vi "Periodic Tasks.vi"(8 "error in":errorcluster) -> (0 "error out":errorcluster)   [LabVIEW 2020]
doc: "This VI runs in parallel to other tasks. It can contain as many user-defined periodic loops as you need. These can carry out PID or other sorts of timed response."
uses:
  <vilib>/Rock Robotics/WPI/ThirdParty/Phoenix-LabVIEW/Motor Controller/Controls/CTRE_Phoenix_MotorControl_ControlMode.ctl
  <vilib>/Rock Robotics/WPI/Utilities/WPI_GetSetVariantRefNum.vi
  Robot Global Data.vi
  2018 Power Up/2018 Robot Project V.3.0/Robot Global Data V.3.0.vi
panel:
  out "Dart Run Speed":dbl
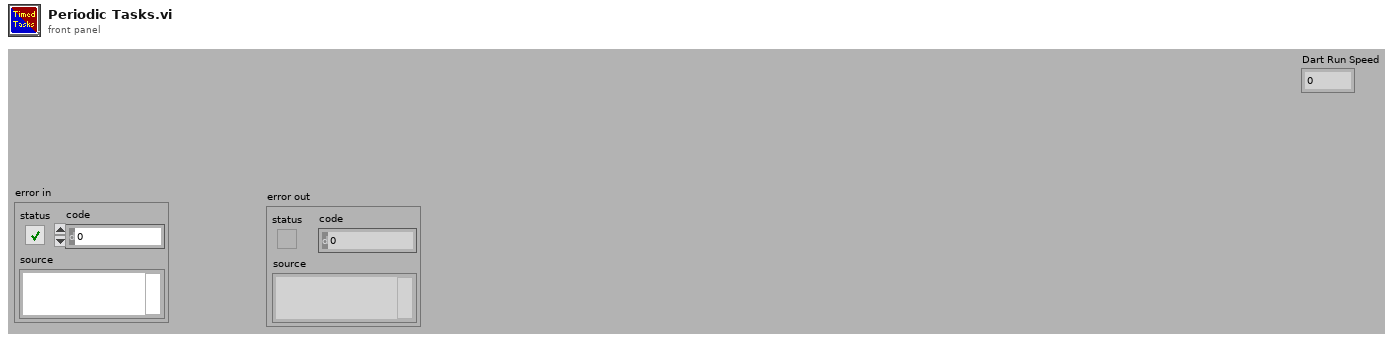
[diagram p1: front panel]
types:
  T1 = typedef "WPI_CounterDevRef.ctl" = cluster{"DevStatus":errorcluster, "CntIndex":T2}
  T2 = typedef "FPGA_CounterCtrSystemIndex.ctl" = enum8{"Ctr 0", "Ctr 1", "Ctr 2", "Ctr 3", "Ctr 4", "Ctr 5", "Ctr 6", "Ctr 7", "Invalid"}
  T3 = typedef "WPI_JoystickDevRef.ctl" = cluster{"Device":T4}
  T4 = typedef "WPI_JoystickDeviceEnum.ctl" = enum16{"USB 0", "USB 1", "USB 2", "USB 3", "USB 4", "USB 5"}
  T5 = typedef "WPI_ServoDeviceRef.ctl" = cluster{"DeviceStatus":errorcluster, "PWM Channel":T6, "DeadBand":T7}
  T6 = typedef "FPGA_DIOPWMChannel.ctl" = enum8{"PWM 0", "PWM 1", "PWM 2", "PWM 3", "PWM 4", "PWM 5", "PWM 6", "PWM 7", "PWM 8", "PWM 9", "PWM MXP 0", "PWM MXP 1", "PWM MXP 2", "PWM MXP 3", "PWM MXP 4", "PWM MXP 5", "PWM MXP 6", "PWM MXP 7", "PWM MXP 8", "PWM MXP 9", "Invalid"}
  T7 = typedef "WPI_PWMDeadband.ctl" = cluster{"Name":string, "maxPositivePwm":i32, "minPositivePwm":i32, "centerPwm":i32, "maxNegativePwm":i32, "minNegativePwm":i32, "angularRange":u16}
  T8 = typedef "WPI_PotentiometerDevRef.ctl" = cluster{"DevStatus":errorcluster, "Analog Channel":T9, "Invert Output":bool}
  T9 = typedef "FPGA_AIChannel.ctl" = enum8{"AI 0", "AI 1", "AI 2", "AI 3", "AI MXP 0", "AI MXP 1", "AI MXP 2", "AI MXP 3", "Invalid"}
  T10 = typedef "WPI_AnalogChannelDevRef.ctl" = cluster{"DevStatus":errorcluster, "Analog Channel":T9}
  T11 = typedef "WPI_DriverStationRobotMode2.ctl" = enum16{"Autonomous Disabled", "Autonomous Enabled", "Teleop Disabled", "Teleop Enabled", "Disconnected", "Finish", "Test Disabled", "Test Enabled", "Emergency Stopped"}
  T12 = typedef "WPI_MotorControlDeviceRef.ctl" = cluster{"DeviceStatus":errorcluster, "Type":T13, "PWM":cluster{"PWM Channel":T6, "DeadBand":T7}, "CAN":cluster{"Device Number":u8, "SetOutput VI Ref":variant, "GetOutput VI Ref":variant, "Enable VI Ref":variant, "Disable VI Ref":variant, "Data":variant}, "Invert":bool, "DIO PWM":cluster{"PWM \"Enable\" Channel":T6, "DIOChannel":T14, "PWM Rate":dbl}}
  T13 = typedef "WPI_MotorControlType.ctl" = enum16{"PWM", "CAN", "DIO PWM"}
  T14 = typedef "FPGA_DIOChannel.ctl" = enum8{"DIO 0", "DIO 1", "DIO 2", "DIO 3", "DIO 4", "DIO 5", "DIO 6", "DIO 7", "DIO 8", "DIO 9", "DIO MXP 0", "DIO MXP 1", "DIO MXP 2", "DIO MXP 3", "DIO MXP 4", "DIO MXP 5", "DIO MXP 6", "DIO MXP 7", "DIO MXP 8", "DIO MXP 9", "DIO MXP 10", "DIO MXP 11", "DIO MXP 12", "DIO MXP 13", "DIO MXP 14", "DIO MXP 15", "SPI Port CS1", "SPI Port CS2", "SPI Port CS3", "SPI Port MISO", "SPI Port MOSI", "Invalid"}
  T15 = typedef "CTRE_Phoenix_MotorControl_ControlMode.ctl" = u16
  T16 = cluster{"Pot. Voltage":dbl[], "Corresponding Inches":dbl[]}
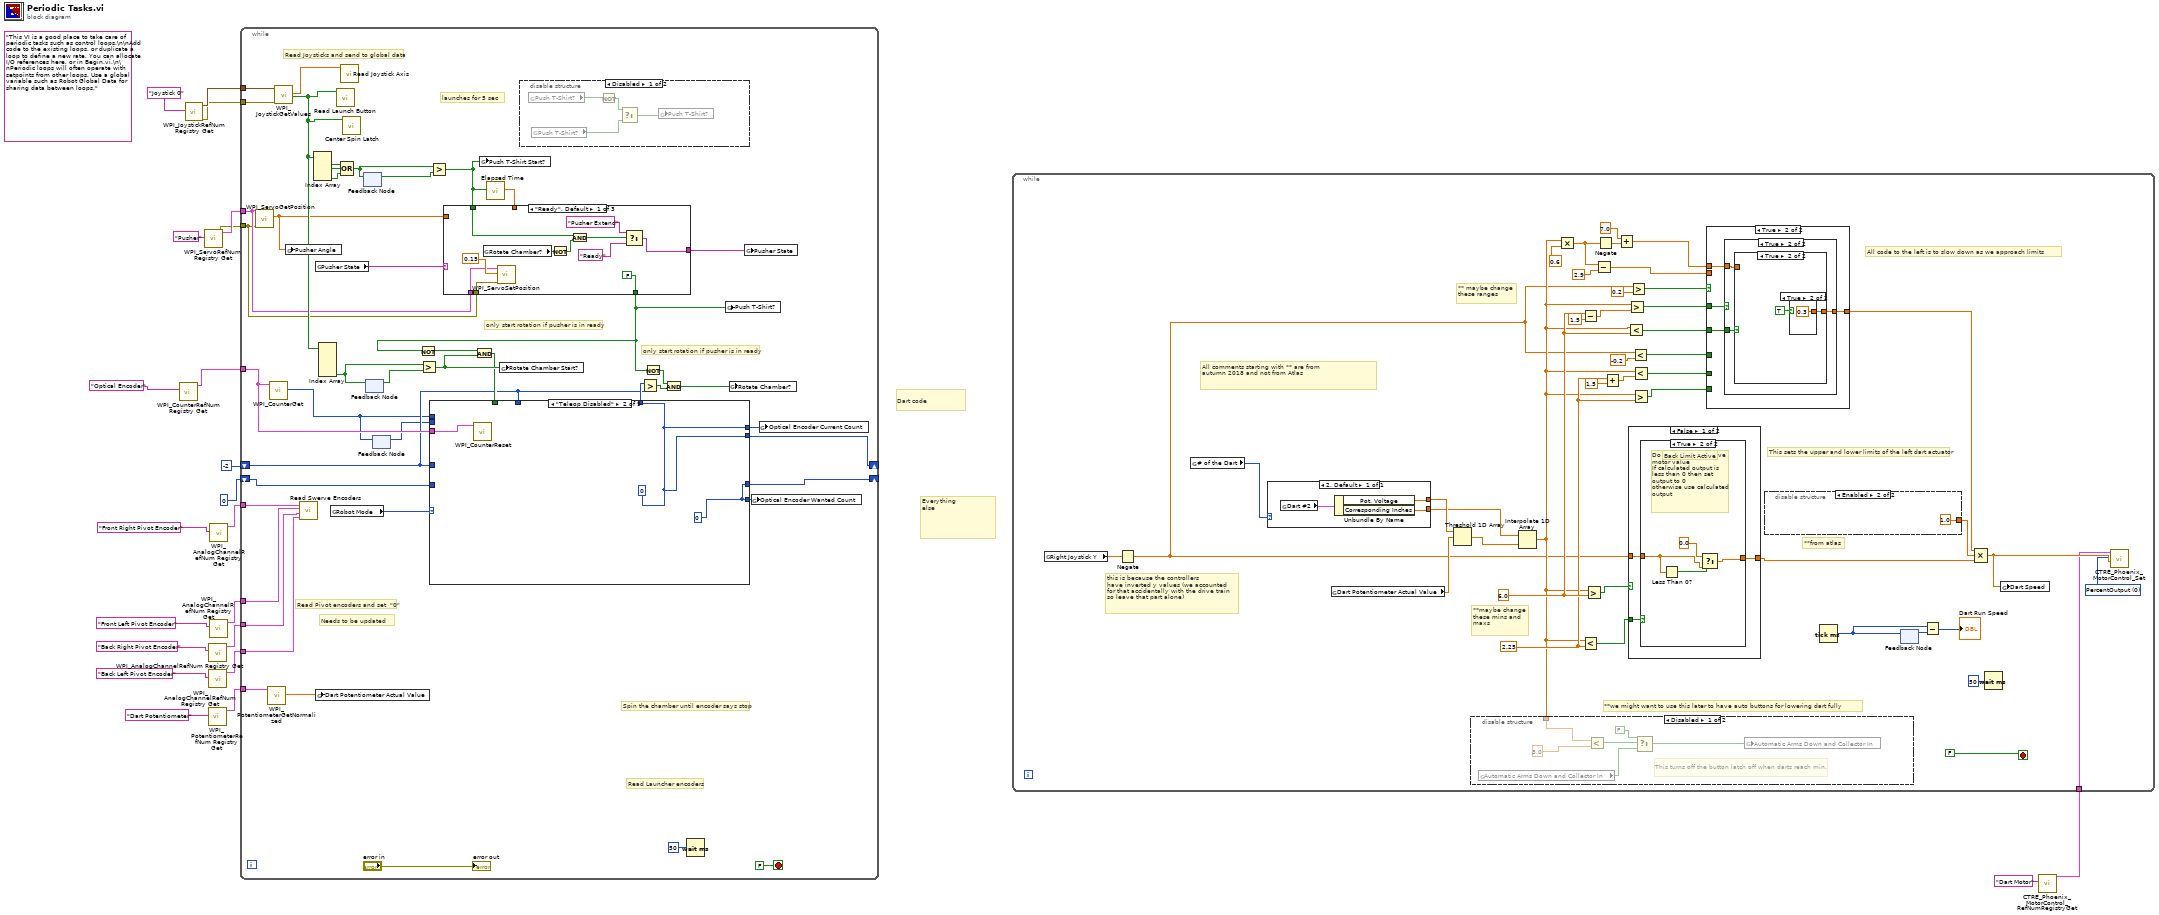
[diagram p0: block diagram]
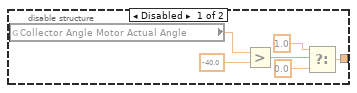
[diagram p2: hidden frame]
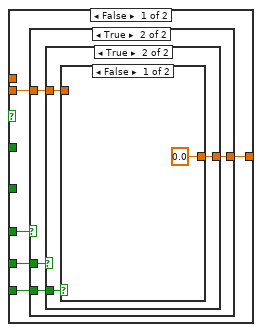
[diagram p4: hidden frame]
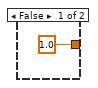
[diagram p5: hidden frame]
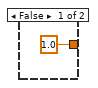
[diagram p6: hidden frame]
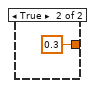
[diagram p7: hidden frame]
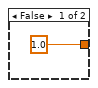
[diagram p8: hidden frame]
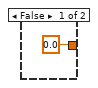
[diagram p9: hidden frame]
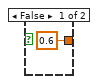
[diagram p10: hidden frame]
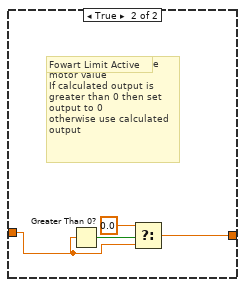
[diagram p12: hidden frame]
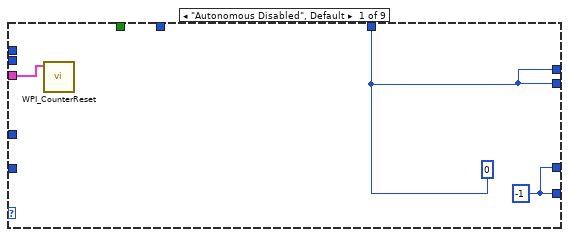
[diagram p13: hidden frame]
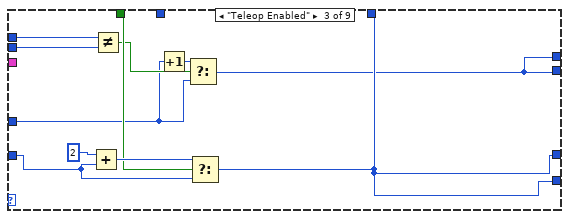
[diagram p14: hidden frame]
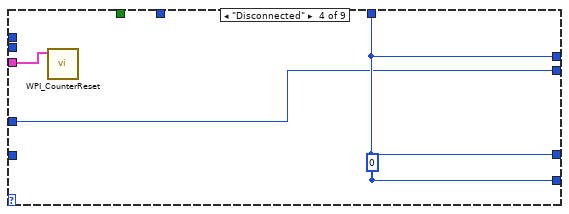
[diagram p15: hidden frame]
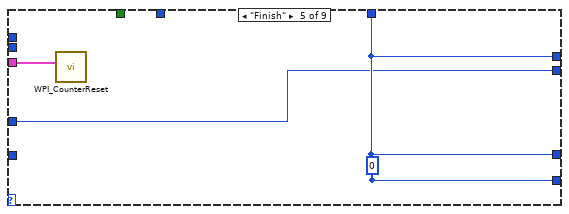
[diagram p16: hidden frame]
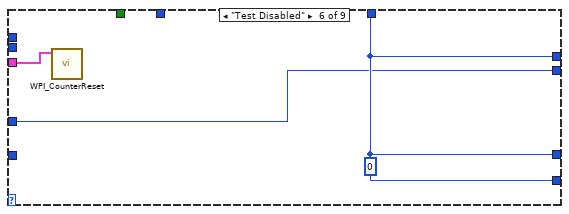
[diagram p17: hidden frame]
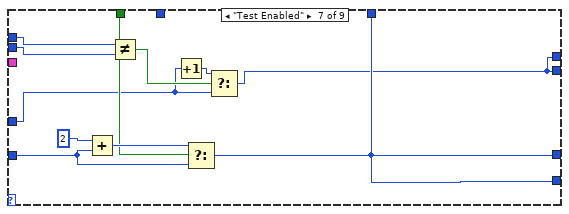
[diagram p18: hidden frame]
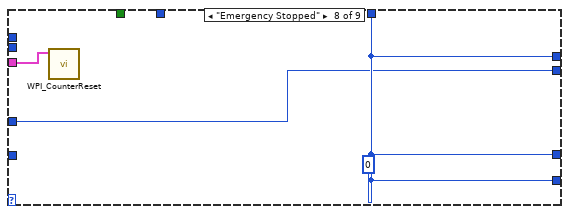
[diagram p19: hidden frame]
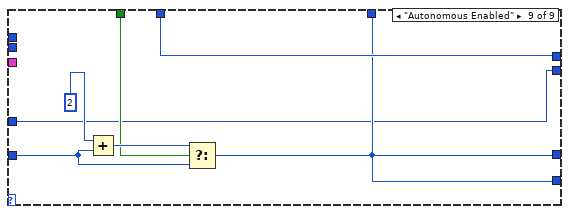
[diagram p20: hidden frame]
diagram:
  (unwired) "This VI is a good place to take care of periodic tasks such as control loops.\n\nAdd code to the existing loops, or duplicate a loop to define a new rate. You can allocate I/O references here, or in Begin.vi.\n\nPeriodic loops will often operate with setpoints from other loops. Use a global variable such as Robot Global Data for sharing data between loops."
  # "Everything\nelse"
  # "Dart code"
  n1 = call <vilib>:"WPI_CounterRefNum Registry Get.vi"("refnum name"="Optical Encoder") -> ("CounterDevRef"=w12:T1)  [unwired: 9 in, 1 out]
  n2 = call <vilib>:"WPI_JoystickRefNum Registry Get.vi"("refnum name"="Joystick 0") -> ("error out"=w20:errorcluster, "JoystickDevRef"=w21:T3)  [unwired: 9 in]
  n3 = call <vilib>:"WPI_ServoRefNum Registry Get.vi"("refnum name"="Pusher") -> ("error out"=w7:errorcluster, "ServoDeviceRef"=w8:T5)  [unwired: 9 in]
  n4 = call <vilib>:"WPI_PotentiometerRefNum Registry Get.vi"("refnum name"="Dart Potentiometer") -> ("PotDevRef"=w4:T8)  [unwired: 9 in, 1 out]
  n5 = call <vilib>:"WPI_AnalogChannelRefNum Registry Get.vi"("refnum name"="Back Right Pivot Encoder") -> ("AIDeviceRef"=w14:T10)  [unwired: 1 in, 9 out]
  n6 = call <vilib>:"WPI_AnalogChannelRefNum Registry Get.vi"("refnum name"="Back Left Pivot Encoder") -> ("AIDeviceRef"=w9:T10)  [unwired: 1 in, 9 out]
  n7 = call <vilib>:"WPI_AnalogChannelRefNum Registry Get.vi"("refnum name"="Front Left Pivot Encoder") -> ("AIDeviceRef"=w15:T10)  [unwired: 1 in, 9 out]
  n8 = call <vilib>:"WPI_AnalogChannelRefNum Registry Get.vi"("refnum name"="Front Right Pivot Encoder") -> ("AIDeviceRef"=w18:T10)  [unwired: 1 in, 9 out]
  n9 = while {
    tunnel: w21 -> [w66]
    tunnel: w20 -> [w65]
    tunnel: w18 -> [w61]
    tunnel: w15 -> [w60]
    tunnel: w14 -> [w59]
    tunnel: w12 -> [w27]
    shift-right: [w33] -> _
    shift-left: 0 -> [w29]
    tunnel: w9 -> [w57]
    tunnel: w8 -> [w51]
    tunnel: w7 -> [w50]
    tunnel: w4 -> [w41]
    shift-right: [w26] -> _
    shift-left: -2 -> [w25]
    stop <- FALSE stop-if-true
    # "only start rotation if pusher is in ready"
    # "only start rotation if pusher is in ready"
    # "Needs to be updated"
    # "launches for 5 sec"
    # "Read Launcher encoders"
    # "Read Pivot encoders and set  \"0\""
    # "Spin the chamber until encoder says stop"
    # "Read Joysticks and send to global data"
    n10 = call <vilib>:"WPI_ServoGetPosition.vi"("error in (no error)"=w50, "ServoDeviceRef"=w51) -> ("Position"=w52:dbl)  [unwired: 7 in, 2 out]
    n11 = call <vilib>:"WPI_PotentiometerGetNormalized.vi"("PotDevRef"=w41) -> ("Normalized Value"=w40:dbl)  [unwired: 8 in, 2 out]
    n12 = call <vilib>:"WPI_CounterGet.vi"("CounterDevRef in"=w27) -> ("Value"=w23:i32)  [unwired: 5 in, 5 out]
    n13 = call <vilib>:"WPI_JoystickGetValues.vi"("error in (no error)"=w65, "JoystickDevRef"=w66) -> ("Buttons"=w56:bool[], "Axes"=w62:dbl[])  [unwired: 5 in, 3 out]
    n14 = global write "Robot Global Data.vi" "Pusher Angle"(w52) -> ()
    n15 = call "Read Swerve Encoders.vi"("BL Ref"=w57, "BR Ref"=w59, "FL Ref"=w60, "FR Ref"=w61) -> ()  [unwired: 1 in]
    n16 = Index Array(array=w56) -> (element #1=w38:bool, element #2=w37:bool, element #4=w36:bool)  [unwired: 4 in, 1 out]
    n17 = global read "Robot Global Data.vi" "Pusher State"() -> (w54:string)
    n18 = global write "Robot Global Data.vi" "Dart Potentiometer Actual Value"(w40) -> ()
    n19 = Index Array(array=w56) -> (element #5=w39:bool)  [unwired: 5 in, 4 out]
    n20 = global read "Robot Global Data.vi" "Robot Mode"() -> (w34:T11)
    n21 = call "Read Launch Button.vi"("array"=w56) -> ()  [unwired: 11 in]
    n22 = call "Read Joystick Axis.vi"("Joystick 0"=w62) -> ()  [unwired: 11 in]
    n23 = Compound Arithmetic op=OR(w38, w37, w36) -> (w35:bool)
    n24 = call "Center Spin Latch.vi"("array"=w56) -> ()  [unwired: 11 in]
    n25 = feedback #1() -> (w55:bool)  [unwired: 1 in]
    n26 = feedback-in #1(w35) -> ()
    n27 = feedback-in #2(w39) -> ()
    n28 = feedback #2() -> (w58:bool)  [unwired: 1 in]
    n29 = feedback #3() -> (w24:i32)  [unwired: 1 in]
    n30 = feedback-in #3(w23) -> ()
    n31 = Greater?(x=w39, y=w58) -> (0:w42:bool)
    n32 = Greater?(x=w35, y=w55) -> (0:w49:bool)
    n33 = global write "Robot Global Data.vi" "Push T-Shirt Start?"(w49) -> ()
    n34 = call "Elapsed Time"("Reset"=w49) -> ("Elapsed Time (s)"=w48:dbl)  [unwired: 11 in, 7 out]
    n35 = case shown="\"Ready\", Default" w54 {
      tunnel: w49 -> [w121 _ _]
      tunnel: [w128 w139 w146] -> w53
      tunnel: w52 -> [_ _ _]
      tunnel: w51 -> [w124 w138 w147]
      tunnel: w50 -> [w125 w135 w145]
      tunnel: [FALSE TRUE TRUE] -> w43
      tunnel: w48 -> [_ w131 w141]
      frame "Ready", Default {
        n36 = global read "Robot Global Data.vi" "Rotate Chamber?"() -> (w123:bool)
        n37 = call <vilib>:"WPI_ServoSetPosition.vi"("error in (no error)"=w125, "Position"=0.15, "ServoDeviceRef"=w124) -> ()  [unwired: 7 in, 2 out]
        n38 = Not(x=w123) -> (.not. x?=w122:bool)
        n39 = And(x=w121, y=w122) -> (x .and. y?=w120:bool)
        n40 = Select(t="Pusher Extend", s=w120, f="Ready") -> (s? t:f=w128:string)
      }
      frame "Pusher Extend" {
        n41 = call <vilib>:"WPI_ServoSetPosition.vi"("error in (no error)"=w135, "Position"=0.9, "ServoDeviceRef"=w138) -> ()  [unwired: 7 in, 2 out]
        n42 = Greater Or Equal?(x=w131, y=5.0) -> (x >= y?=w132:bool)
        n43 = Select(t="Pusher Retract", s=w132, f="Pusher Extend") -> (s? t:f=w139:string)
      }
      frame "Pusher Retract" {
        n44 = call <vilib>:"WPI_ServoSetPosition.vi"("error in (no error)"=w145, "Position"=0.15, "ServoDeviceRef"=w147) -> ()  [unwired: 7 in, 2 out]
        n45 = Greater Or Equal?(x=w141, y=10.0) -> (x >= y?=w142:bool)
        n46 = Select(t="Ready", s=w142, f="Pusher Retract") -> (s? t:f=w146:string)
      }
    }
    n47 = Not(x=w43) -> (.not. x?=w44:bool)
    n48 = And(x=w44, y=w42) -> (x .and. y?=w30:bool)
    n49 = case shown="\"Teleop Disabled\"" w34 {
      tunnel: w29 -> [_ _ w81 _ _ _ w101 _ w111]
      tunnel: [w68 w71 w80 w86 w89 w92 w102 w106 w110] -> w33
      tunnel: [w68 w71 w80 w86 w89 w92 w102 w106 w110] -> w32
      tunnel: [w69 w72 w76 w86 w89 w92 w96 w106 w112] -> w31
      tunnel: w30 -> [_ _ w82 _ _ _ w103 _ w113]
      tunnel: w25 -> [_ _ _ _ _ _ _ _ w112]
      tunnel: [w69 w72 w80 w86 w89 w92 w102 w106 w110] -> w28
      tunnel: w27 -> [w70 w73 _ w87 w90 w93 _ w107 _]
      tunnel: w25 -> [_ _ w78 w85 w88 w91 w97 w105 w108]
      tunnel: [w69 w72 w76 w85 w88 w91 w96 w105 w108] -> w26
      tunnel: w23 -> [_ _ w75 _ _ _ w95 _ _]
      tunnel: w24 -> [_ _ w74 _ _ _ w94 _ _]
      frame "Autonomous Disabled", Default {
        w68 = -1
        w69 = 0
        n50 = call <vilib>:"WPI_CounterReset.vi"("CounterDevRef in"=w70) -> ()  [unwired: 9 in, 2 out]
      }
      frame "Teleop Disabled" {
        w71 = 0
        w72 = 0
        n51 = call <vilib>:"WPI_CounterReset.vi"("CounterDevRef in"=w73) -> ()  [unwired: 9 in, 2 out]
      }
      frame "Teleop Enabled" {
        n52 = Add(x=2, y=w81) -> (x+y=w84:i32)
        n53 = Not Equal?(x=w75, y=w74) -> (x != y?=w79:bool)
        n54 = Increment(x=w78) -> (x+1=w77:i32)
        n55 = Select(t=w77, s=w79, f=w78) -> (s? t:f=w76:i32)
        n56 = Select(t=w84, s=w82, f=w81) -> (s? t:f=w80:i32)
      }
      frame "Disconnected" {
        w86 = 0
        n57 = call <vilib>:"WPI_CounterReset.vi"("CounterDevRef in"=w87) -> ()  [unwired: 9 in, 2 out]
      }
      frame "Finish" {
        w89 = 0
        n58 = call <vilib>:"WPI_CounterReset.vi"("CounterDevRef in"=w90) -> ()  [unwired: 9 in, 2 out]
      }
      frame "Test Disabled" {
        w92 = 0
        n59 = call <vilib>:"WPI_CounterReset.vi"("CounterDevRef in"=w93) -> ()  [unwired: 9 in, 2 out]
      }
      frame "Test Enabled" {
        n60 = Add(x=2, y=w101) -> (x+y=w104:i32)
        n61 = Not Equal?(x=w95, y=w94) -> (x != y?=w99:bool)
        n62 = Increment(x=w97) -> (x+1=w98:i32)
        n63 = Select(t=w104, s=w103, f=w101) -> (s? t:f=w102:i32)
        n64 = Select(t=w98, s=w99, f=w97) -> (s? t:f=w96:i32)
      }
      frame "Emergency Stopped" {
        w106 = 0
        n65 = call <vilib>:"WPI_CounterReset.vi"("CounterDevRef in"=w107) -> ()  [unwired: 9 in, 2 out]
      }
      frame "Autonomous Enabled" {
        n66 = Add(x=2, y=w111) -> (x+y=w114:i32)
        n67 = Select(t=w114, s=w113, f=w111) -> (s? t:f=w110:i32)
      }
    }
    n68 = global write "Robot Global Data.vi" "Rotate Chamber Start?"(w42) -> ()
    n69 = disable-structure shown="Disabled" {
      frame Disabled {
        n70 = global read "Robot Global Data.vi" "Push T-Shirt?"() -> (w115:bool)
        n71 = global read "Robot Global Data.vi" "Push T-Shirt?"() -> (w117:bool)
        n72 = Not(x=w115) -> (.not. x?=w116:bool)
        n73 = Select(t=w116, f=w117) -> (s=w119:bool, s? t:f=w118:bool)
        n74 = global write "Robot Global Data.vi" "Push T-Shirt?"(w118) -> ()
      }
      frame Enabled {
      }
    }
    n75 = Greater?(x=w28, y=w25) -> (0:w46:bool)
    n76 = Not(x=w43) -> (.not. x?=w45:bool)
    n77 = And(x=w45, y=w46) -> (x .and. y?=w47:bool)
    n78 = Wait (ms)(milliseconds to wait=50) -> ()  [unwired: 1 out]
    n79 = global write "Robot Global Data.vi" "Push T-Shirt?"(w43) -> ()
    n80 = global write "Robot Global Data.vi" "Rotate Chamber?"(w47) -> ()
    n81 = global write "Robot Global Data.vi" "Pusher State"(w53) -> ()
    n82 = global write "Robot Global Data.vi" "Optical Encoder Wanted Count"(w32) -> ()
    n83 = global write "Robot Global Data.vi" "Optical Encoder Current Count"(w31) -> ()
    "error out" <- "error in"
  }
  n84 = call <vilib>:"CTRE_Phoenix_MotorControl_RefNumRegistryGet.vi"("refnum name"="Dart Motor") -> ("PhoenixMotorControlDevRef"=w2:T12)  [unwired: 9 in, 1 out]
  n85 = while {
    tunnel: w2 -> [w153]
    stop <- FALSE stop-if-true
    w151 = T15 0 items=["PercentOutput"=0, "Position"=1, "Velocity"=2, "Current"=3, "Follower"=5, "MotionProfile"=6, "MotionMagic"=7, "MotionProfileArc"=10, "Disabled"=15] ("Control Mode")
    w162 = 2.25 ("x")
    w166 = 6.0 ("x")
    # "this is because the controllers\nhave inverted y values (we accounted\nfor that accidentally with the drive train\nso leave that part alone)"
    # "** maybe change\nthese ranges"
    # "All comments starting with ** are from \nautumn 2018 and not from Atlas"
    # "**maybe change\nthese mins and \nmaxs"
    # "**from atlas"
    # "**we might want to use this later to have auto buttons for lowering dart fully"
    # "All code to the left is to slow down as we approach limits"
    # "This sets the upper and lower limits of the left dart actuator"
    n86 = global read "Robot Global Data.vi" "Right Joystick Y"() -> (w155:dbl)
    n87 = Negate(x=w155) -> (-x=w152:dbl)
    n88 = global read "Robot Global Data.vi" "# of the Dart"() -> (w184:i32)
    n89 = case shown="2, Default" w184 {
      tunnel: [w236] -> w186
      tunnel: [w235] -> w185
      frame 2, Default {
        n90 = global read "Robot Global Data.vi" "Dart #2"() -> (w237:T16)
        n91 = Unbundle By Name(w237) -> ("Pot. Voltage"=w236:dbl[], "Corresponding Inches"=w235:dbl[])
      }
    }
    n92 = global read "Robot Global Data.vi" "Dart Potentiometer Actual Value"() -> (w187:dbl)
    n93 = Threshold 1D Array(2:w187, 3:w186) -> (0:w188:dbl)  [unwired: 1 in]
    n94 = Interpolate 1D Array(1:w188, 2:w185) -> (0:w156:dbl)
    n95 = disable-structure shown="Disabled" {
      disable-tunnel: w156 -> [w200 _]
      frame Disabled {
        # "This turns off the button latch off when darts reach min."
        n96 = global read "Robot Global Data V.3.0.vi" "Automatic Arms Down and Collector In"() -> (w201:bool)
        n97 = Less?(x=w200, y=3.0 ("x")) -> (x < y?=w204:bool)
        n98 = Select(t=FALSE, s=w204, f=w201) -> (s? t:f=w203:bool)
        n99 = global write "Robot Global Data V.3.0.vi" "Automatic Arms Down and Collector In"(w203) -> ()
      }
      frame Enabled {
      }
    }
    n100 = Multiply(x=w156, y=0.6) -> (x*y=w176:dbl)
    n101 = Subtract(x=w166, y=1.5) -> (x-y=w164:dbl)
    n102 = Less?(x=w156, y=w162) -> (x < y?=w189:bool)
    n103 = Greater?(x=w156, y=w166) -> (0:w190:bool)
    n104 = Subtract(x=w176, y=2.9) -> (x-y=w167:dbl)
    n105 = Negate(x=w176) -> (-x=w178:dbl)
    n106 = Add(x=w162, y=1.5) -> (x+y=w163:dbl)
    n107 = Add(x=7.0, y=w178) -> (x+y=w171:dbl)
    n108 = Less?(x=w156, y=w166) -> (x < y?=w172:bool)
    n109 = Greater?(x=w156, y=w164) -> (0:w173:bool)
    n110 = case shown="False" w190 {
      tunnel: [w240 w248] -> w183
      tunnel: w152 -> [w239 w246]
      tunnel: w189 -> [w238 _]
      frame False {
        n111 = case shown="True" w238 {
          tunnel: [w241 w243] -> w240
          tunnel: w239 -> [w241 w242]
          frame False {
            # "Use calculate\nvalue"
            # "No Limits Active"
          }
          frame True {
            # "Do not allow a negitive\nmotor value\nIf calculated output is\nless than 0 then set\noutput to 0\notherwise use calculated\noutput"
            # "Back Limit Active"
            n112 = Less Than 0?(x=w242) -> (x < 0?=w245:bool)
            n113 = Select(t=0.0, s=w245, f=w242) -> (s? t:f=w243:dbl)
          }
        }
      }
      frame True {
        # "Do not allow a positive\nmotor value\nIf calculated output is\ngreater than 0 then set\noutput to 0\notherwise use calculated\noutput"
        # "Fowart Limit Active"
        n114 = Greater Than 0?(x=w246) -> (x > 0?=w249:bool)
        n115 = Select(t=0.0, s=w249, f=w246) -> (s? t:f=w248:dbl)
      }
    }
    n116 = Greater?(x=w152, y=0.2) -> (0:w174:bool)
    n117 = Less?(x=w152, y=-0.2) -> (x < y?=w170:bool)
    n118 = Less?(x=w156, y=w163) -> (x < y?=w169:bool)
    n119 = Greater?(x=w156, y=w162) -> (0:w168:bool)
    n120 = case shown="True" w174 {
      tunnel: w173 -> [_ w225]
      tunnel: w172 -> [_ w224]
      tunnel: w171 -> [_ w223]
      tunnel: [w209 w222] -> w157
      tunnel: w170 -> [w210 _]
      tunnel: w169 -> [w208 _]
      tunnel: w168 -> [w207 _]
      tunnel: w167 -> [w206 _]
      frame False {
        n121 = case shown="True" w210 {
          tunnel: [1.0 w214] -> w209
          tunnel: w208 -> [_ w215]
          tunnel: w207 -> [_ w213]
          tunnel: w206 -> [_ w212]
          frame False {
          }
          frame True {
            n122 = case shown="True" w215 {
              tunnel: [1.0 w218] -> w214
              tunnel: w213 -> [_ w219]
              tunnel: w212 -> [_ w217]
              frame False {
              }
              frame True {
                n123 = case shown="False" w219 {
                  tunnel: [0.0 0.3] -> w218
                  tunnel: w217 -> [_ _]
                  frame False {
                  }
                  frame True {
                  }
                }
              }
            }
          }
        }
      }
      frame True {
        n124 = case shown="True" w225 {
          tunnel: w224 -> [_ w229]
          tunnel: w223 -> [_ w228]
          tunnel: [1.0 w227] -> w222
          frame False {
          }
          frame True {
            n125 = case shown="True" w229 {
              tunnel: w228 -> [_ _]
              tunnel: [0.0 w232] -> w227
              frame False {
              }
              frame True {
                n126 = case shown="True" TRUE {
                  tunnel: [0.6 0.3] -> w232
                  frame False {
                  }
                  frame True {
                  }
                }
              }
            }
          }
        }
      }
    }
    n127 = disable-structure shown="Enabled" {
      disable-tunnel: [w193 1.0] -> w158
      frame Disabled {
        n128 = global read "Robot Global Data V.3.0.vi" "Collector Angle Motor Actual Angle"() -> (w198:dbl)
        n129 = Greater?(x=w198, y=-40.0) -> (0:w196:bool)
        n130 = Select(t=1.0, s=w196, f=0.0) -> (s? t:f=w193:dbl)
      }
      frame Enabled {
      }
    }
    n131 = Tick Count (ms)() -> (millisecond timer value=w181:u32)
    n132 = feedback #4() -> (w182:u32)  [unwired: 1 in]
    n133 = feedback-in #4(w181) -> ()
    n134 = Subtract(x=w181, y=w182) -> (x-y=→"Dart Run Speed":u32)
    n135 = Compound Arithmetic op=MULTIPLY(w157, w158, w183) -> (w154:dbl)
    n136 = Wait (ms)(milliseconds to wait=u32 50) -> ()  [unwired: 1 out]
    n137 = global write "Robot Global Data.vi" "Dart Speed"(w154) -> ()
    n138 = call <vilib>:"CTRE_Phoenix_MotorControl_Set.vi"("Output"=w154, "Control Mode"=w151, "PhoenixMotorControlDevRef"=w153) -> ()  [unwired: 7 in, 2 out]
  }
